vi "example async wait for stop.vi"() -> ()   [LabVIEW 2016]
panel:
  in  "System Locator":string="usb:ix:0"
  in  "Delta Steps":i32[](array[numeric])=[50000, -100000, 200000, -400000]
  in  "stop":bool
  out "Error":errorcluster
  in  "Channel":u32
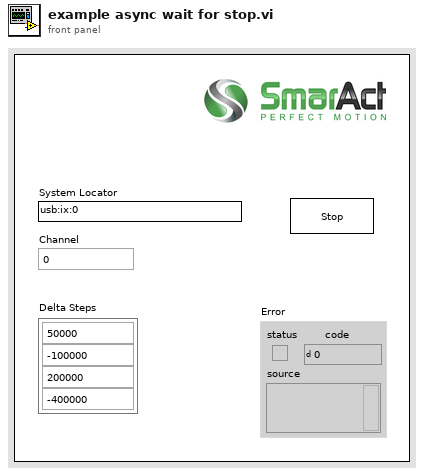
[diagram p1: front panel]
types:
  T1 = enum32{"SA_SENSOR_DISABLED", "SA_SENSOR_ENABLED", "SA_SENSOR_POWERSAVE"}
  T2 = enum32{"SA_UNBUFFERED_OUTPUT", "SA_BUFFERED_OUTPUT"}
  T3 = typedef "mcsPacket.ctl" = cluster{"packetType":enum32{"SA_NO PACKET_TYPE", "SA_ERROR_ PACKET_TYPE", "SA_POSITION PACKET_TYPE", "SA_COMPLETED PACKET_TYPE", "SA_STATUS PACKET_TYPE", "SA_ANGLE_PACKET_TYPE", "SA_VOLTAGE_LEVEL_PACKET_TYPE", "SA_SENSOR_TYPE_PACKET_TYPE", "SA_SENSOR_ENABLED_PACKET_TYPE", "SA_END_EFFECTOR_TYPE_PACKET_TYPE", "SA_GRIPPER_OPENING_PACKET_TYPE", "SA_FORCE_PACKET_TYPE", "SA_MOVE_SPEED_PACKET_TYPE", "SA_PHYSICAL_POSITION_KNOWN_PACKET_TYPE", "SA_POSITION_LIMIT_PACKET_TYPE", "SA_ANGLE_LIMIT_PACKET_TYPE", "SA_SAFE_DIRECTION_PACKET_TYPE", "SA_SCALE_PACKET_TYPE", "SA_MOVE_ACCELERATION_PACKET_TYPE", "SA_CHANNEL_PROPERTY_PACKET_TYPE", "SA_CAPTURE_BUFFER_PACKET_TYPE", "SA_TRIGGERED_PACKET_TYPE"}, "channelIndex":u32, "data1":u32, "data2":i32, "data3":i32, "data4":u32}
  T4 = enum32{"SA_NO PACKET_TYPE", "SA_ERROR_ PACKET_TYPE", "SA_POSITION PACKET_TYPE", "SA_COMPLETED PACKET_TYPE", "SA_STATUS PACKET_TYPE", "SA_ANGLE_PACKET_TYPE", "SA_VOLTAGE_LEVEL_PACKET_TYPE", "SA_SENSOR_TYPE_PACKET_TYPE", "SA_SENSOR_ENABLED_PACKET_TYPE", "SA_END_EFFECTOR_TYPE_PACKET_TYPE", "SA_GRIPPER_OPENING_PACKET_TYPE", "SA_FORCE_PACKET_TYPE", "SA_MOVE_SPEED_PACKET_TYPE", "SA_PHYSICAL_POSITION_KNOWN_PACKET_TYPE", "SA_POSITION_LIMIT_PACKET_TYPE", "SA_ANGLE_LIMIT_PACKET_TYPE", "SA_SAFE_DIRECTION_PACKET_TYPE", "SA_SCALE_PACKET_TYPE", "SA_MOVE_ACCELERATION_PACKET_TYPE", "SA_CHANNEL_PROPERTY_PACKET_TYPE", "SA_CAPTURE_BUFFER_PACKET_TYPE", "SA_TRIGGERED_PACKET_TYPE"}
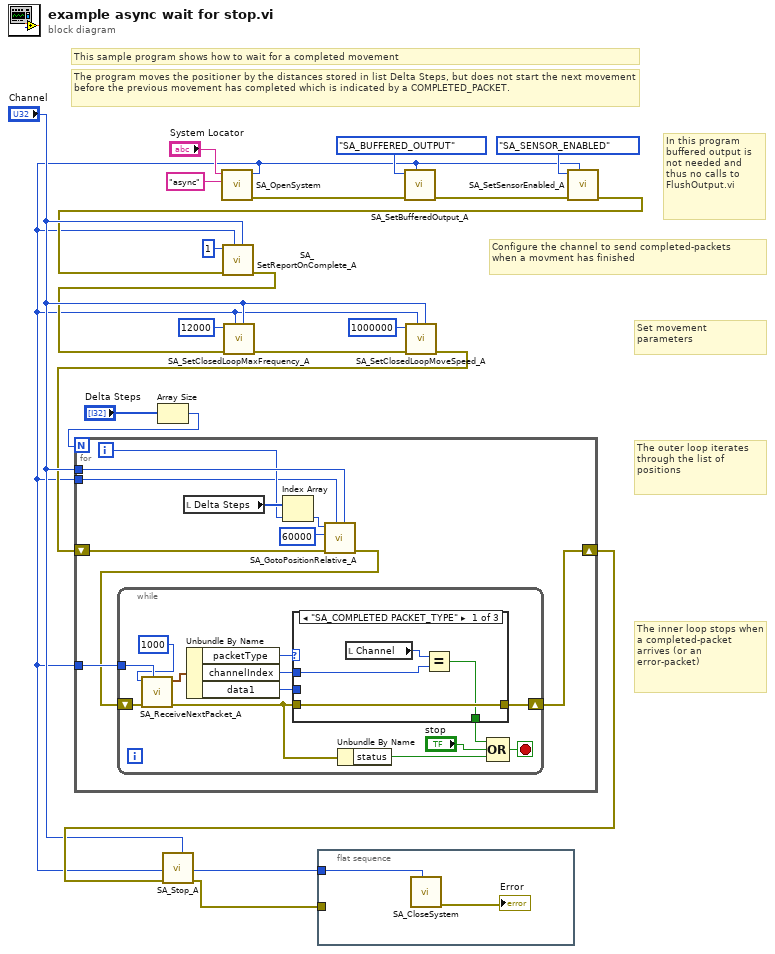
[diagram p0: block diagram]
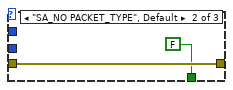
[diagram p2: hidden frame]
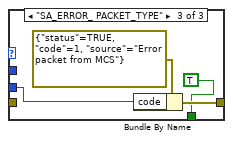
[diagram p3: hidden frame]
diagram:
  # "In this program buffered output is not needed and thus no calls to FlushOutput.vi"
  # "Set movement parameters"
  # "The program moves the positioner by the distances stored in list Delta Steps, but does not start the next movement before the previous movement has completed which is indicated by a COMPLETED_PACKET."
  # "The outer loop iterates through the list of positions"
  # "The inner loop stops when a completed-packet arrives (or an error-packet)"
  # "This sample program shows how to wait for a completed movement"
  # "Configure the channel to send completed-packets\nwhen a movment has finished"
  n1 = Array Size(array="Delta Steps") -> (size(s)=w15:i32)
  n2 = call <vilib>:"SA_OpenSystem.vi"("options"="async", "systemLocator"="System Locator") -> ("error out"=w19:errorcluster, "systemIndexOut"=w2:u32)  [unwired: 8 in]
  n3 = flat-sequence {
    tunnel: w2 -> [w20]
    tunnel: w1 -> [_]
    frame #0 {
      n4 = call <vilib>:"SA_CloseSystem.vi"("systemIndex"=w20) -> ("error out"=→"Error":errorcluster)  [unwired: 10 in]
    }
  }
  n5 = call <vilib>:"SA_SetBufferedOutput_A.vi"("systemIndex"=w2, "error in (no error)"=w19, "mode"=T2."SA_BUFFERED_OUTPUT") -> ("error out"=w7:errorcluster)  [unwired: 8 in]
  n6 = call <vilib>:"SA_SetSensorEnabled_A.vi"("systemIndex"=w2, "error in (no error)"=w7, "enabled"=T1."SA_SENSOR_ENABLED") -> ("error out"=w6:errorcluster)  [unwired: 8 in]
  n7 = call <vilib>:"SA_SetReportOnComplete_A.vi"("channelIndex"="Channel", "systemIndex"=w2, "error in (no error)"=w6, "report"=u32 1 ("systemIndex")) -> ("error out"=w8:errorcluster)  [unwired: 7 in]
  n8 = call <vilib>:"SA_SetClosedLoopMaxFrequency_A.vi"("channelIndex"="Channel", "systemIndex"=w2, "error in (no error)"=w8, "frequency"=u32 12000) -> ("error out"=w12:errorcluster)  [unwired: 7 in]
  n9 = call <vilib>:"SA_SetClosedLoopMoveSpeed_A.vi"("channelIndex"="Channel", "systemIndex"=w2, "error in (no error)"=w12, "speed"=u32 1000000) -> ("error out"=w5:errorcluster)  [unwired: 7 in]
  n10 = for {
    N: w15 -> [_]
    tunnel: w2 -> [w31]
    tunnel: "Channel" -> [w30]
    tunnel: w2 -> [w23]
    shift-right: [w27] -> w16
    shift-left: w5 -> [w29]
    i -> [w24]
    n11 = local read "Delta Steps"() -> (w25:i32[])
    n12 = Index Array(array=w25, index=w24) -> (element=w26:i32)
    n13 = call <vilib>:"SA_GotoPositionRelative_A.vi"("channelIndex"=w30, "systemIndex"=w23, "error in (no error)"=w29, "holdTime"=u32 60000, "diff"=w26) -> ("error out"=w22:errorcluster)  [unwired: 6 in]
    n14 = while {
      tunnel: w31 -> [w44]
      shift-right: [w40] -> w27
      shift-left: w22 -> [w41]
      stop <- w35 stop-if-true
      n15 = call <vilib>:"SA_ReceiveNextPacket_A.vi"("systemIndex"=w44, "error in (no error)"=w41, "timeout"=u32 1000) -> ("error out"=w36:errorcluster, "packet"=w42:T3)  [unwired: 7 in]
      n16 = Unbundle By Name(w42) -> ("packetType"=w37:T4, "channelIndex"=w38:u32, "data1"=w39:u32)
      n17 = case shown="\"SA_COMPLETED PACKET_TYPE\"" w37 {
        tunnel: w36 -> [w48 w50 _]
        tunnel: [w48 w50 w53] -> w40
        tunnel: w39 -> [_ _ w52]
        tunnel: [w47 FALSE TRUE] -> w34
        tunnel: w38 -> [w45 _ _]
        frame "SA_COMPLETED PACKET_TYPE" {
          n18 = local read "Channel"() -> (w46:u32)
          n19 = Equal?(x=w46, y=w45) -> (x = y?=w47:bool)
        }
        frame "SA_NO PACKET_TYPE", Default {
        }
        frame "SA_ERROR_ PACKET_TYPE" {
          n20 = Bundle By Name(cluster=errorcluster {"status"=TRUE, "code"=1, "source"="Error packet from MCS"} ("error out"), "code"=w52) -> (w53:errorcluster)
        }
      }
      n21 = Unbundle By Name(w36) -> ("status"=w32:bool)
      n22 = Compound Arithmetic op=OR(w34, "stop", w32) -> (w35:bool)
    }
  }
  n23 = call <vilib>:"SA_Stop_A.vi"("channelIndex"="Channel", "systemIndex"=w2, "error in (no error)"=w16) -> ("error out"=w1:errorcluster)  [unwired: 8 in]
